vi "Destroy.vi"(8 "error in (no error)":errorcluster, 11 "CIFTemplatePlugin in":refnum<class "TemplatePlugin.lvclass">) -> (0 "error out":errorcluster, 3 "CIFTemplatePlugin out":refnum<class "TemplatePlugin.lvclass">)   [LabVIEW 2021, in "TemplatePlugin.lvclass"]
uses:
  TemplatePlugin.lvclass
  TemplatePlugin.lvclass/TemplatePlugin.ctl
  OOB/OOB_Tx/TemplateOOB_Tx.lvclass
  D:/dev/CIF-LVCore/src/CIFUtilities/CIFOutOfBand/CIFOutOfBand.lvclass
  OOB/OOB_Rx/TemplateOOB_Rx.lvclass
  CIF-LVCore/src/CIFUtilities/CIFOutOfBand/CIFOutOfBand.lvclass
  D:/dev/Plugins/Template/OOB/OOB_Rx/TemplateOOB_Rx.lvclass
  D:/dev/Plugins/Template/OOB/OOB_Tx/TemplateOOB_Tx.lvclass
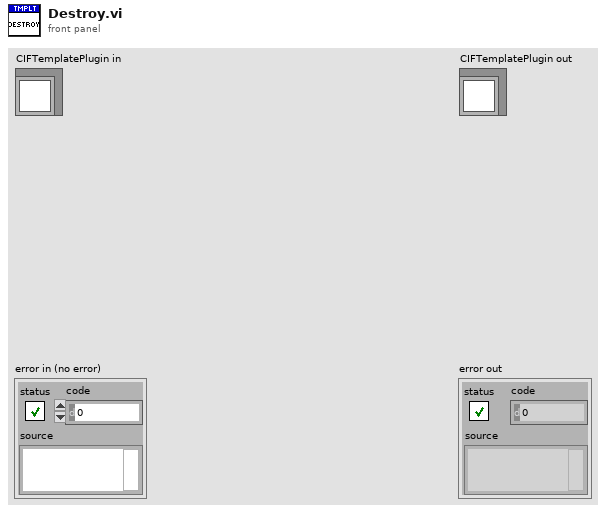
[diagram p1: front panel]
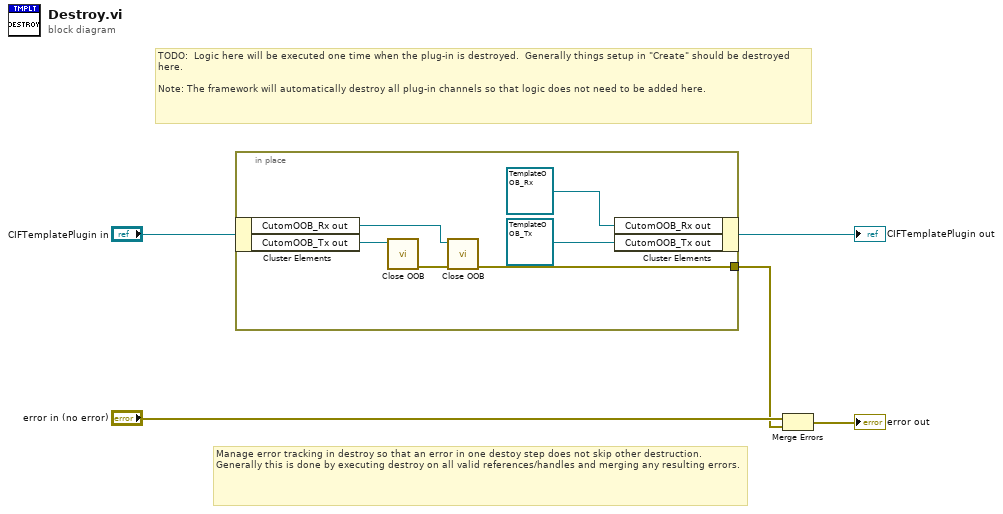
[diagram p0: block diagram]
diagram:
  # "TODO:  Logic here will be executed one time when the plug-in is destroyed.  Generally things setup in \"Create\" should be destroyed here.  \n\nNote: The framework will automatically destroy all plug-in channels so that logic does not need to be added here."
  # "Manage error tracking in destroy so that an error in one destoy step does not skip other destruction.   Generally this is done by executing destroy on all valid references/handles and merging any resulting errors."
  n1 = in-place {
    in-place-border: [w6] -> w1
    n2 = in-place-cluster #1("CIFTemplatePlugin in") -> ("CutomOOB_Rx out"=w10:refnum<class "TemplateOOB_Rx.lvclass">, "CutomOOB_Tx out"=w11:refnum<class "TemplateOOB_Tx.lvclass">)
    n3 = call "Close OOB.vi"("OOB in"=w11) -> ("error out"=w9:errorcluster)  [unwired: 10 in]
    n4 = call "Close OOB.vi"("error in"=w9, "OOB in"=w10) -> ("error out"=w6:errorcluster)  [unwired: 9 in]
    n5 = in-place-cluster #1("CutomOOB_Rx out"=refnum<class "TemplateOOB_Rx.lvclass"> refnum, "CutomOOB_Tx out"=refnum<class "TemplateOOB_Tx.lvclass"> refnum) -> (→"CIFTemplatePlugin out":refnum<class "TemplatePlugin.lvclass">)
  }
  n6 = Merge Errors("error in (no error)", w1) -> (→"error out":errorcluster)
